vi "PID Process Value and Error_NONREENTRANT.vi"(6 "PID Config":T1={"Gains"={"P"=1.0, "I"=0.01, "D"=0.0, "F"=0.0}, "Error Allowed"={"High"=0.1, "Low"=-0.1}, "I Zone"={"High"=10.0, "Low"=-10.0}, "Max Out"={"FWD"=100.0, "REV"=-100.0}, "Max I Accu"={"High"=0.0, "Low"=0.0}, "CL Ramp Rate (S)"=0.0} {"Max I Accu"."Low" format="%#.8f"; "Max I Accu"."High" format="%#.8f"; "Gains"."F" format="%#.8f"; "Gains"."D" format="%#.8f"; "Gains"."I" format="%#.8f"; "Gains"."P" format="%#.8f"; "Error Allowed"."Low" format="%#.8f"; "Error Allowed"."High" format="%#.8f"; "I Zone"."Low" format="%#.8f"; "I Zone"."High" format="%#.8f"; "Max Out"."REV" format="%.2f"; "Max Out"."FWD" format="%.2f"}, 7 "Target Cycle Time(S)":dbl=0.05 format="%.3f", 8 "Allowable Error Disables Accumulator":bool=TRUE, 9 "ERROR":dbl format="%.2f", 11 "Process Variable":dbl format="%.2f") -> (0 "PID Enabled Out":bool, 1 "I Accumulator":dbl, 2 "Error Out":dbl, 3 "Output Out":dbl format="%.2f", 5 "Time Mulitplyer Out":dbl)   [LabVIEW 2020]
uses:
  Shared Code/TypeDefs/Cluster_PID Config.ctl
  Shared Code/TypeDefs/Cluster_PID Gains.ctl
  Shared Code/TypeDefs/Cluster_High-Low.ctl
  Shared Code/TypeDefs/Cluster_FWD  REV Values.ctl
  <vilib>/addons/control/pid/NI_PID_pid.lvlib
  <vilib>/addons/control/pid/pid.llb/PID (DBL).vi
panel:
  out "In Izone":bool
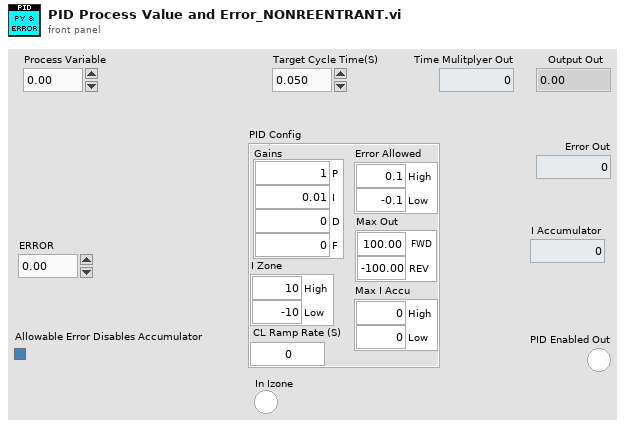
[diagram p1: front panel]
types:
  T1 = typedef "Cluster_PID Config.ctl" = cluster{"Gains":T2, "Error Allowed":T3, "I Zone":T3, "Max Out":T4, "Max I Accu":T3, "CL Ramp Rate (S)":dbl}
  T2 = typedef "Cluster_PID Gains.ctl" = cluster{"P":dbl, "I":dbl, "D":dbl, "F":dbl}
  T3 = typedef "Cluster_High-Low.ctl" = cluster{"High":dbl, "Low":dbl}
  T4 = typedef "Cluster_FWD  REV Values.ctl" = cluster{"FWD":dbl, "REV":dbl}
  T5 = cluster{"PID gains":T2, "error":dbl, "process variable":dbl, "output ":dbl, "derivative action":dbl, "I Accumulator":dbl, "Previous Time":dbl, "Same Gains":bool, "time mulitplyer":dbl, "previous error":dbl, "Propotional Action":dbl, "Previous Process Value":dbl, "PID Enabled":bool, "PID Config":T1, "FeedForward Action":dbl, "Allowable Error Disables Accumulator":bool, "Current Time":dbl}
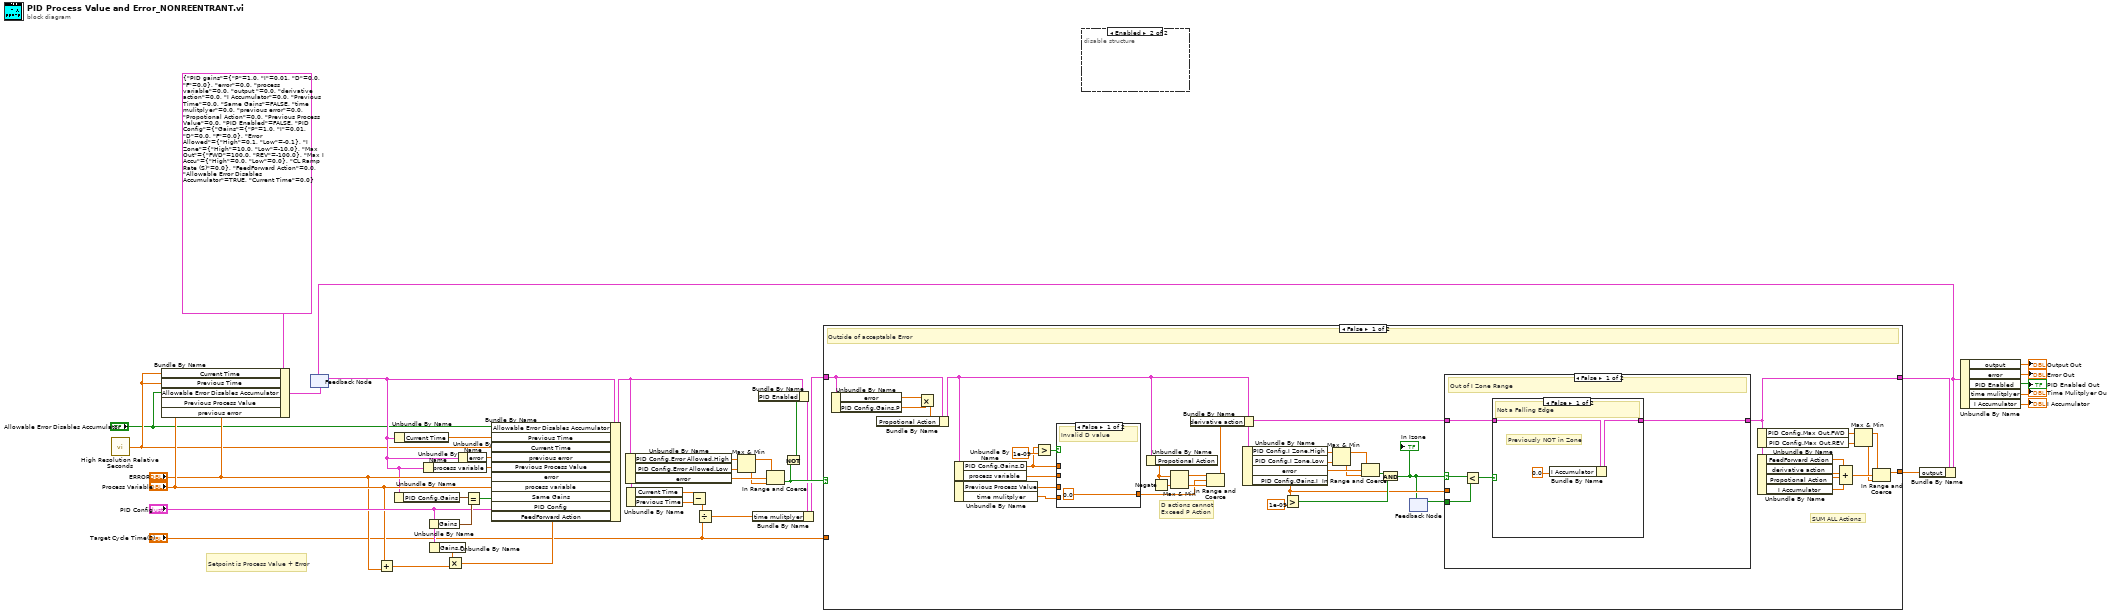
[diagram p0: block diagram]
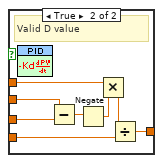
[diagram p2: hidden frame]
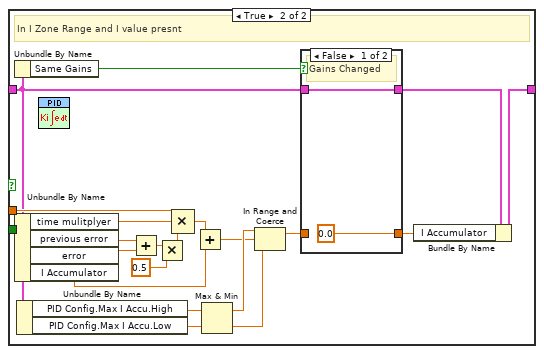
[diagram p4: hidden frame]
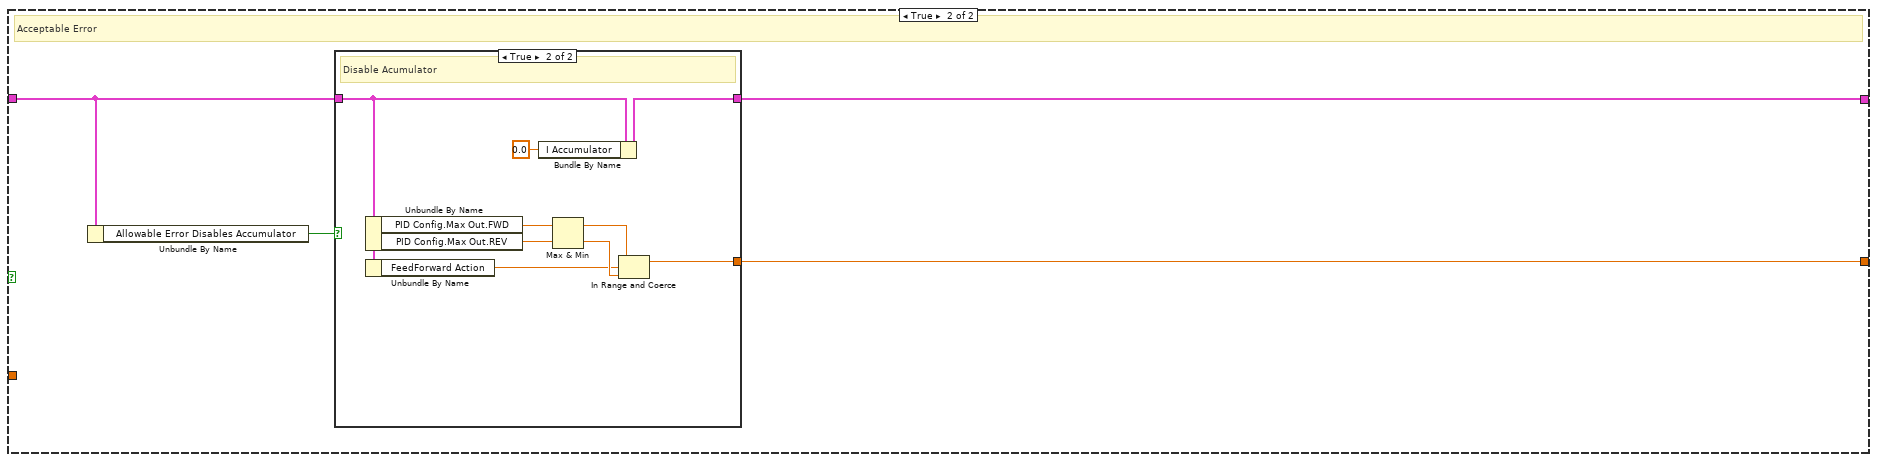
[diagram p6: hidden frame]
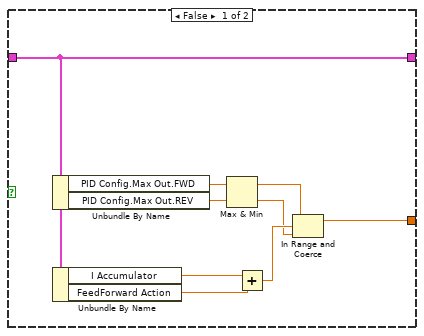
[diagram p7: hidden frame]
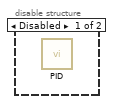
[diagram p8: hidden frame]
diagram:
  # "Setpoint is Process Value + Error"
  n1 = call <vilib>:"High Resolution Relative Seconds.vi"() -> ("relative seconds"=w11:dbl)
  n2 = Bundle By Name(cluster=T5 {"PID gains"={"P"=1.0, "I"=0.01, "D"=0.0, "F"=0.0}, "error"=0.0, "process variable"=0.0, "output "=0.0, "derivative action"=0.0, "I Accumulator"=0.0, "Previous Time"=0.0, "Same Gains"=FALSE, "time mulitplyer"=0.0, "previous error"=0.0, "Propotional Action"=0.0, "Previous Process Value"=0.0, "PID Enabled"=FALSE, "PID Config"={"Gains"={"P"=1.0, "I"=0.01, "D"=0.0, "F"=0.0}, "Error Allowed"={"High"=0.1, "Low"=-0.1}, "I Zone"={"High"=10.0, "Low"=-10.0}, "Max Out"={"FWD"=100.0, "REV"=-100.0}, "Max I Accu"={"High"=0.0, "Low"=0.0}, "CL Ramp Rate (S)"=0.0}, "FeedForward Action"=0.0, "Allowable Error Disables Accumulator"=TRUE, "Current Time"=0.0} ("Keep  Cluster"), "Current Time"=w11, "Previous Time"=w11, "Allowable Error Disables Accumulator"="Allowable Error Disables Accumulator", "Previous Process Value"="Process Variable", "previous error"="ERROR") -> (w26:T5)
  n3 = feedback #1(w26) -> (w13:T5)
  n4 = Add(x="Process Variable", y="ERROR") -> (x+y=w15:dbl)
  n5 = Unbundle By Name(w13) -> ("PID Config.Gains"=w21:T2)
  n6 = Unbundle By Name(w13) -> ("Current Time"=w12:dbl)
  n7 = Unbundle By Name(w13) -> ("process variable"=w34:dbl)
  n8 = Unbundle By Name("PID Config") -> ("Gains"=w23:T2)
  n9 = Unbundle By Name("PID Config") -> ("Gains.F"=w19:dbl)
  n10 = Multiply(x=w19, y=w15) -> (x*y=w14:dbl)
  n11 = Unbundle By Name(w13) -> ("error"=w35:dbl)
  n12 = Equal?(x=w21, y=w23) -> (x = y?=w22:bool)
  n13 = Bundle By Name(cluster=w13, "Allowable Error Disables Accumulator"="Allowable Error Disables Accumulator", "Previous Time"=w12, "Current Time"=w11, "previous error"=w35, "Previous Process Value"=w34, "error"="ERROR", "process variable"="Process Variable", "Same Gains"=w22, "PID Config"="PID Config", "FeedForward Action"=w14) -> (w4:T5)
  n14 = Unbundle By Name(w4) -> ("PID Config.Error Allowed.High"=w32:dbl, "PID Config.Error Allowed.Low"=w31:dbl, "error"=w33:dbl)
  n15 = Unbundle By Name(w4) -> ("Current Time"=w6:dbl, "Previous Time"=w7:dbl)
  n16 = Subtract(x=w6, y=w7) -> (x-y=w5:dbl)
  n17 = Divide(x=w5, y="Target Cycle Time(S)") -> (x/y=w2:dbl)
  n18 = Max & Min(x=w32, y=w31) -> (max(x,y)=w29:dbl, min(x,y)=w30:dbl)
  n19 = In Range and Coerce(upper limit=w29, x=w33, lower limit=w30) -> (In Range?=w28:bool)  [unwired: 1 out]
  n20 = Not(x=w28) -> (.not. x?=w27:bool)
  n21 = Bundle By Name(cluster=w4, "PID Enabled"=w27) -> (w9:T5)
  n22 = Bundle By Name(cluster=w9, "time mulitplyer"=w2) -> (w8:T5)
  n23 = case shown="False" w28 {
    tunnel: [w63 w125] -> w24
    tunnel: "Target Cycle Time(S)" -> [_ _]
    tunnel: w8 -> [w45 w124]
    tunnel: [w62 w126] -> w18
    frame False {
      # "SUM ALL Actions"
      # "D actions cannot\nExceed P Action"
      # "Outside of acceptable Error"
      n24 = Unbundle By Name(w45) -> ("error"=w78:dbl, "PID Config.Gains.P"=w77:dbl)
      n25 = Multiply(x=w78, y=w77) -> (x*y=w75:dbl)
      n26 = Bundle By Name(cluster=w45, "Propotional Action"=w75) -> (w44:T5)
      n27 = Unbundle By Name(w44) -> ("PID Config.Gains.D"=w58:dbl, "process variable"=w79:dbl)
      n28 = Unbundle By Name(w44) -> ("Previous Process Value"=w80:dbl, "time mulitplyer"=w43:dbl)
      n29 = Greater?(x=w58, y=1e-09) -> (0:w59:bool)
      n30 = case shown="False" w59 {
        tunnel: w80 -> [_ w87]
        tunnel: w43 -> [_ w86]
        tunnel: w79 -> [_ w84]
        tunnel: [0.0 w85] -> w53
        tunnel: w58 -> [_ w82]
        frame False {
          # "Invalid D value"
        }
        frame True {
          # "Valid D value"
          n31 = Subtract(x=w84, y=w87) -> (x-y=w89:dbl)
          n32 = Negate(x=w89) -> (-x=w83:dbl)
          n33 = Multiply(x=w82, y=w83) -> (x*y=w88:dbl)
          n34 = Divide(x=w88, y=w86) -> (x/y=w85:dbl)
        }
      }
      n35 = Unbundle By Name(w44) -> ("Propotional Action"=w57:dbl)
      n36 = Negate(x=w57) -> (-x=w56:dbl)
      n37 = Max & Min(x=w57, y=w56) -> (max(x,y)=w55:dbl, min(x,y)=w54:dbl)
      n38 = In Range and Coerce(upper limit=w55, x=w53, lower limit=w54) -> (coerced(x)=w52:dbl)  [unwired: 1 out]
      n39 = Bundle By Name(cluster=w44, "derivative action"=w52) -> (w76:T5)
      n40 = Unbundle By Name(w44) -> ("PID Config.I Zone.High"=w69:dbl, "PID Config.I Zone.Low"=w68:dbl, "error"=w74:dbl, "PID Config.Gains.I"=w70:dbl)
      n41 = Greater?(x=w70, y=1e-09) -> (0:w71:bool)
      n42 = Max & Min(x=w69, y=w68) -> (max(x,y)=w66:dbl, min(x,y)=w67:dbl)
      n43 = In Range and Coerce(upper limit=w66, x=w74, lower limit=w67) -> (In Range?=w73:bool)  [unwired: 1 out]
      n44 = And(x=w73, y=w71) -> (x .and. y?=w42:bool)
      "In Izone" <- w42
      n45 = feedback-in #2(w42) -> ()
      n46 = feedback #2() -> (w41:bool)  [unwired: 1 in]
      n47 = case shown="False" w42 {
        selector: w42 -> [w92 _]
        tunnel: [w94 w101] -> w63
        tunnel: w76 -> [w93 w104]
        tunnel: w70 -> [_ w111]
        tunnel: w41 -> [w91 _]
        frame False {
          # "Out of I Zone Range"
          n48 = Less?(x=w92, y=w91) -> (x < y?=w90:bool)
          n49 = case shown="False" w90 {
            tunnel: [w97 w98] -> w94
            tunnel: w93 -> [w96 w98]
            frame False {
              # "Previously NOT in Zone"
              # "Not a Falling Edge"
              n50 = Bundle By Name(cluster=w96, "I Accumulator"=0.0) -> (w97:T5)
            }
            frame True {
              # "Previously in Zone"
              # "Falling Edge"
            }
          }
        }
        frame True {
          # "In I Zone Range and I value presnt"
          n51 = Unbundle By Name(w104) -> ("Same Gains"=w110:bool)
          n52 = Unbundle By Name(w104) -> ("time mulitplyer"=w117:dbl, "previous error"=w116:dbl, "error"=w115:dbl, "I Accumulator"=w109:dbl)
          n53 = Unbundle By Name(w104) -> ("PID Config.Max I Accu.High"=w106:dbl, "PID Config.Max I Accu.Low"=w105:dbl)
          n54 = Add(x=w116, y=w115) -> (x+y=w114:dbl)
          n55 = Multiply(x=w114, y=0.5) -> (x*y=w112:dbl)
          n56 = Compound Arithmetic op=MULTIPLY(w111, w117, w112) -> (w118:dbl)
          n57 = Add(x=w118, y=w109) -> (x+y=w103:dbl)
          n58 = Max & Min(x=w106, y=w105) -> (max(x,y)=w108:dbl, min(x,y)=w107:dbl)
          n59 = In Range and Coerce(upper limit=w108, x=w103, lower limit=w107) -> (coerced(x)=w102:dbl)  [unwired: 1 out]
          n60 = case shown="False" w110 {
            tunnel: w102 -> [_ w122]
            tunnel: [0.0 w122] -> w99
            tunnel: w104 -> [w120 w121]
            tunnel: [w120 w121] -> w100
            frame False {
              # "Gains Changed"
            }
            frame True {
              # "Reinitialize or Same Gains"
            }
          }
          n61 = Bundle By Name(cluster=w100, "I Accumulator"=w99) -> (w101:T5)
        }
      }
      n62 = Unbundle By Name(w63) -> ("PID Config.Max Out.FWD"=w49:dbl, "PID Config.Max Out.REV"=w48:dbl)
      n63 = Unbundle By Name(w63) -> ("FeedForward Action"=w51:dbl, "derivative action"=w64:dbl, "Propotional Action"=w65:dbl, "I Accumulator"=w50:dbl)
      n64 = Compound Arithmetic op=ADD(w51, w64, w65, w50) -> (w61:dbl)
      n65 = Max & Min(x=w49, y=w48) -> (max(x,y)=w46:dbl, min(x,y)=w47:dbl)
      n66 = In Range and Coerce(upper limit=w46, x=w61, lower limit=w47) -> (coerced(x)=w62:dbl)  [unwired: 1 out]
    }
    frame True {
      # "Acceptable Error"
      n67 = Unbundle By Name(w124) -> ("Allowable Error Disables Accumulator"=w123:bool)
      n68 = case shown="True" w123 {
        tunnel: [w135 w144] -> w126
        tunnel: w124 -> [w127 w138]
        tunnel: [w127 w139] -> w125
        frame False {
          n69 = Unbundle By Name(w127) -> ("PID Config.Max Out.FWD"=w133:dbl, "PID Config.Max Out.REV"=w132:dbl)
          n70 = Unbundle By Name(w127) -> ("I Accumulator"=w129:dbl, "FeedForward Action"=w128:dbl)
          n71 = Max & Min(x=w133, y=w132) -> (max(x,y)=w130:dbl, min(x,y)=w131:dbl)
          n72 = Add(x=w129, y=w128) -> (x+y=w134:dbl)
          n73 = In Range and Coerce(upper limit=w130, x=w134, lower limit=w131) -> (coerced(x)=w135:dbl)  [unwired: 1 out]
        }
        frame True {
          # "Disable Acumulator"
          n74 = Unbundle By Name(w138) -> ("PID Config.Max Out.FWD"=w143:dbl, "PID Config.Max Out.REV"=w142:dbl)
          n75 = Unbundle By Name(w138) -> ("FeedForward Action"=w136:dbl)
          n76 = Bundle By Name(cluster=w138, "I Accumulator"=0.0) -> (w139:T5)
          n77 = Max & Min(x=w143, y=w142) -> (max(x,y)=w140:dbl, min(x,y)=w141:dbl)
          n78 = In Range and Coerce(upper limit=w140, x=w136, lower limit=w141) -> (coerced(x)=w144:dbl)  [unwired: 1 out]
        }
      }
    }
  }
  n79 = disable-structure shown="Enabled" {
    frame Disabled {
      n80 = call-poly <vilib>:"PID.vi"() -> ()  [unwired: 10 in, 2 out]
    }
    frame Enabled {
    }
  }
  n81 = Bundle By Name(cluster=w24, "output"=w18) -> (w25:T5)
  n82 = feedback-in #1(w25) -> ()
  n83 = Unbundle By Name(w25) -> ("output"=→"Output Out":dbl, "error"=→"Error Out":dbl, "PID Enabled"=→"PID Enabled Out":bool, "time mulitplyer"=→"Time Mulitplyer Out":dbl, "I Accumulator"=→"I Accumulator":dbl)
